vi "WindSensorSignature.vi"(11 "WindSensorSignatureSettings":T1={"DataFIFO"="InclinometerRxCRCFIFO", "CalculateFIFO"="InclinometerCalculateCRCFIFO", "SignatureFIFO"="InclinometerCalculatedCRCFIFO"}) -> ()   [LabVIEW 2018]
uses:
  WindSensorSignatureSettings.ctl
  WindSensorSignatureData.ctl
  WindSensorSignatureStates.ctl
  <vilib>/Platform/TimedLoop/XDataNode/timing_clust.ctl
  <vilib>/Platform/TimedLoop/XDataNode/nitl_modes.ctl
  <vilib>/Platform/TimedLoop/XDataNode/wakeup.ctl
  <vilib>/rvi/Emulation/niFpgaSctlEmulationGetInTimedLoop.vi
  <vilib>/rvi/Emulation/niFpgaEmulationReportErrorSimple.vi
  <vilib>/rvi/Emulation/niFpgaGetClockAttributes.vi
  <vilib>/rvi/Emulation/niFpgaCriticalErrorInLSC.vi
  <vilib>/rvi/DataTransferAndStorage/Container/Common/niFpgaContainerExecOnDevCompGetState.vi
  <vilib>/rvi/Emulation/niFpgaEmulationIsFPGAContextNoSignature.vi
  <vilib>/rvi/errors/niFpgaSetErrorForExecOnDevCompSimple.vi
  <vilib>/rvi/eio/common/nirviEmuReportErrorAndStop.vi
  <vilib>/rvi/DataTransferAndStorage/Container/Common/niFpgaContainerGetUniqueNameForEmu.vi
  <vilib>/rvi/FIFO/Fifo_Resource/nirvififoEmulationSetSize.vi
  <vilib>/rvi/FIFO/Fifo_Resource/nirviFifoEmulationQueueMgr.vi
  <instcachedir>/0/nirviFifoEmulationQueueMgr_E5CAEC123FF24DC58D834DCA3CDAA9B5.lvgen/nirviFifoEmulationQueueMgr_E5CAEC123FF24DC58D834DCA3CDAA9B5_001.vi
  <vilib>/rvi/FIFO/Fifo_Resource/nirvififoEmulationDetermineInputValidOut.vi
  <vilib>/rvi/FIFO/Fifo_Resource/nirvififoEmulationCreateLock.vi
  <vilib>/rvi/Emulation/niFpgaProcessEmulError.vi
  <vilib>/rvi/FIFO/Fifo_Resource/nirvififoEmulationObtainLock.vi
  <vilib>/rvi/FIFO/Fifo_Resource/nirvififoEmulationReleaseLock.vi
  <vilib>/rvi/occurrence/nirviWaitOnOccurrenceBase.vi
  <vilib>/rvi/errors/nirviReportUnexpectedCaseInternalError.vi
  <vilib>/rvi/errors/nirviReportUnexpectedCaseInternalError (U32).vi
  <vilib>/Utility/error.llb/Clear Errors.vi
  <vilib>/rvi/interface/RandomDataEmulation/niFpgaRandomDataHandleErrors.vi
  <instcachedir>/0/nirviFifoEmulationQueueMgr_E5CAEC123FF24DC58D834DCA3CDAA9B5.lvgen/nirviFifoEmulationQueueMgr_E5CAEC123FF24DC58D834DCA3CDAA9B5_002.vi
  <instcachedir>/0/nirviFifoEmulationQueueMgr_E5CAEC123FF24DC58D834DCA3CDAA9B5.lvgen/nirviFifoEmulationQueueMgr_E5CAEC123FF24DC58D834DCA3CDAA9B5_004.vi
  <vilib>/Platform/TimedLoop/XDataNode/XDataNode.xnode
  <vilib>/rvi/DataTransferAndStorage/Container/XNode/niFpgaContainer.xnode
  <vilib>/rvi/FIFO/Fifo_Resource/niFpgaFifoEmulationRefIn.vi
  <vilib>/Platform/TimedLoop/XDataNode/XDNodeRunTimeDep.lvlib
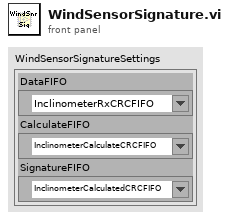
[diagram p1: front panel]
types:
  T1 = typedef "WindSensorSignatureSettings.ctl" = cluster{"DataFIFO":refnum<k21>, "CalculateFIFO":refnum<k21>, "SignatureFIFO":refnum<k21>}
  T2 = typedef "WindSensorSignatureData.ctl" = cluster{"State":T3, "Word":u8, "Signature":u16}
  T3 = typedef "WindSensorSignatureStates.ctl" = enum16{"WaitForData", "ProcessData", "CheckForPublish", "PublishCRC"}
  T4 = typedef "XDNodeRunTimeDep.lvlib/timing_clust.ctl" = cluster{"Expected End [f-1]":u64, "Actual End [f-1]":u64, "Finished Late? [f-1]":bool, "Expected End [i-1]":u64, "Actual End [i-1]":u64, "Finished Late? [i-1]":bool, "Expected Start [i]":u64, "Actual Start [i]":u64, "Expected Start [f]":u64, "Actual Start [f]":u64, "Source Name":string, "Structure Name":string, "Period":i64, "Deadline":i64, "Offset":i64, "Start":i64, "Priority":i32, "Timeout":i32, "Mode":T5, "Wakeup Reason":T6, "Error":errorcluster, "Source Type":string, "Secondary Source Type":string, "Global End Time":u64, "Global Start Time":u64, "Frame Duration":u64, "Iteration Duration":u64, "Assigned CPU":i32, "I/O Scan Engine Mode":u32}
  T5 = typedef "XDNodeRunTimeDep.lvlib/nitl_modes.ctl" = enum32{"No Change", "Process missed periods, maintain original phase", "Discard missed periods, maintain original phase", "Process missed periods, ignore original phase", "Discard missed periods, ignore original phase"}
  T6 = typedef "XDNodeRunTimeDep.lvlib/wakeup.ctl" = enum32{"Normal", "Aborted", "Asynchronous wakeup", "Timing source error", "Timed loop error", "Timeout"}
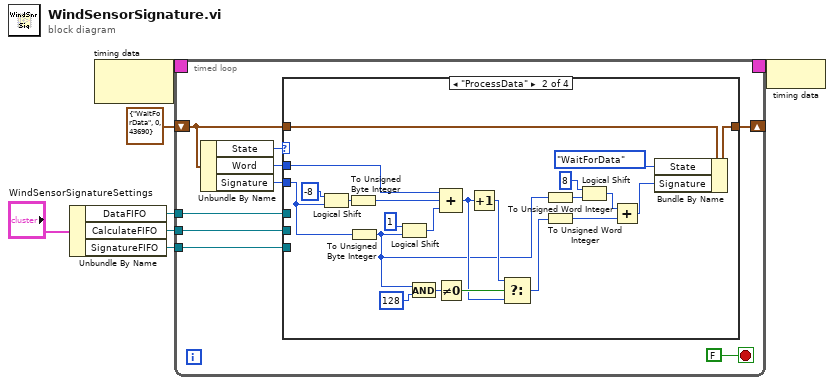
[diagram p0: block diagram]
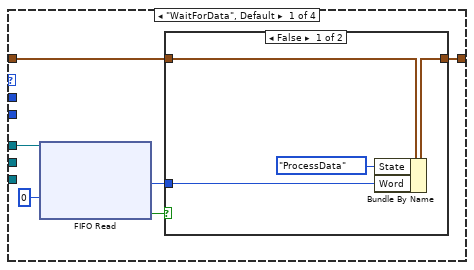
[diagram p2: hidden frame]
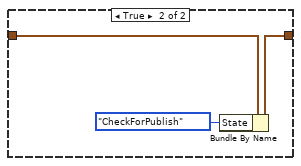
[diagram p3: hidden frame]
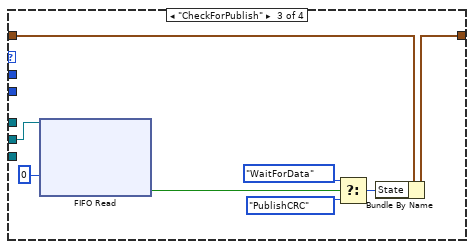
[diagram p4: hidden frame]
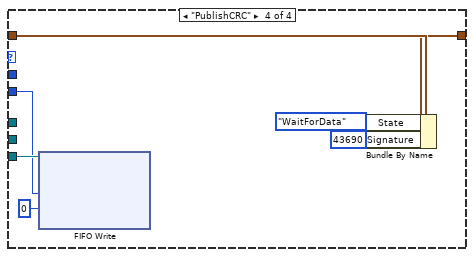
[diagram p5: hidden frame]
diagram:
  n1 = Unbundle By Name("WindSensorSignatureSettings") -> ("DataFIFO"=w3:refnum<k21>, "CalculateFIFO"=w2:refnum<k21>, "SignatureFIFO"=w1:refnum<k21>)
  n2 = node-c288() -> (w6:T4)  [unwired: 1 in]
  n3 = timed-loop {
    shift-right: [w15] -> _
    shift-left: T2 {"State"=enum."WaitForData", "Word"=0, "Signature"=43690} ("ModbusCRCData") -> [w14]
    timing: w6 -> [_]
    timing-out: [_] -> w5
    tunnel: w3 -> [w12]
    tunnel: w2 -> [w11]
    tunnel: w1 -> [w10]
    stop <- FALSE stop-if-true
    n4 = Unbundle By Name(w14) -> ("State"=w16:T3, "Word"=w9:u8, "Signature"=w13:u16)
    n5 = case shown="\"ProcessData\"" w16 {
      tunnel: [w17 w50 w58 w65] -> w15
      tunnel: w14 -> [w22 w51 w59 w66]
      tunnel: w13 -> [_ w49 _ w62]
      tunnel: w12 -> [w21 _ _ _]
      tunnel: w11 -> [_ _ w57 _]
      tunnel: w10 -> [_ _ _ w63]
      tunnel: w9 -> [_ w37 _ _]
      frame "WaitForData", Default {
        n6 = xnode ("FIFO Read")("Timeout"=0, "FIFO In"=w21) -> ("Element"=w18:u8, "Timed Out?"=w19:bool)  [unwired: 1 out]
        n7 = case shown="False" w19 {
          tunnel: w22 -> [w26 w29]
          tunnel: w18 -> [w23 _]
          tunnel: [w25 w28] -> w17
          frame False {
            n8 = Bundle By Name(cluster=w26, "State"=WindSensorSignatureStates."ProcessData", "Word"=w23) -> (w25:T2)
          }
          frame True {
            n9 = Bundle By Name(cluster=w29, "State"=WindSensorSignatureStates."CheckForPublish") -> (w28:T2)
          }
        }
      }
      frame "ProcessData" {
        n10 = Logical Shift(y=i16 -8, x=w49) -> (x << y=w47:u16)
        n11 = To Unsigned Byte Integer(number=w47) -> (unsigned 8bit integer=w38:u8)
        n12 = To Unsigned Byte Integer(number=w49) -> (unsigned 8bit integer=w30:u8)
        n13 = Logical Shift(y=i16 1, x=w30) -> (x << y=w39:u8)
        n14 = And(x=w30, y=u8 128) -> (x .and. y?=w35:u8)
        n15 = Not Equal To 0?(x=w35) -> (x != 0?=w34:bool)
        n16 = Compound Arithmetic op=ADD(w37, w38, w39) -> (w32:u8)
        n17 = Increment(x=w32) -> (x+1=w31:u8)
        n18 = Select(t=w31, s=w34, f=w32) -> (s? t:f=w33:u8)
        n19 = To Unsigned Word Integer(number=w30) -> (unsigned 16bit integer=w43:u16)
        n20 = To Unsigned Word Integer(number=w33) -> (unsigned 16bit integer=w46:u16)
        n21 = Logical Shift(y=i16 8, x=w43) -> (x << y=w45:u16)
        n22 = Add(x=w45, y=w46) -> (x+y=w42:u16)
        n23 = Bundle By Name(cluster=w51, "State"=WindSensorSignatureStates."WaitForData" ("t"), "Signature"=w42) -> (w50:T2)
      }
      frame "CheckForPublish" {
        n24 = xnode ("FIFO Read")("Timeout"=0, "FIFO In"=w57) -> ("Timed Out?"=w55:bool)  [unwired: 2 out]
        n25 = Select(t=WindSensorSignatureStates."WaitForData" ("State"), s=w55, f=WindSensorSignatureStates."PublishCRC" ("State")) -> (s? t:f=w52:T3)
        n26 = Bundle By Name(cluster=w59, "State"=w52) -> (w58:T2)
      }
      frame "PublishCRC" {
        n27 = xnode ("FIFO Write")("Element"=w62, "Timeout"=0, "FIFO In"=w63) -> ()  [unwired: 2 out]
        n28 = Bundle By Name(cluster=w66, "State"=WindSensorSignatureStates."WaitForData", "Signature"=u16 43690 ("CRC")) -> (w65:T2)
      }
    }
  }
  n29 = node-c288(w5) -> ()
